vi "Any_Ref_enthalpy_funct_PS_REFPROP10.vi"(1 "Pressure Out (kPa)":dbl, 2 "S_in":dbl, 3 "error in (no error)":errorcluster, 4 "Fluidofinterest":string="R134a.FLD", 5 "?":path=path "C:/Users/ASITest/Desktop/REFPROP") -> (8 "h2_s":dbl, 10 "error out":errorcluster)   [LabVIEW 2016]
doc: "Return refrigerant enthalpy [kJ/kg] for specified refrigerant, input pressure [kPa] and temperature [C]"
panel:
  out "name out":string
  out "data":string[][](table)=[["0", "T", "40.917420"], ["1", "P", "632.917420"], ["2", "H", "466.332574"], ["3", "S", "2.054657"], ["4", "DV", "18.926081"], ["5", "DL", "18.926081"], ["6", "E", "432.891028"], ["7", "CV", "0.758226"], ["8", "CP", "0.924261"], ["9", "W", "194.299169"], ["10", "Q", "998.000000"]]
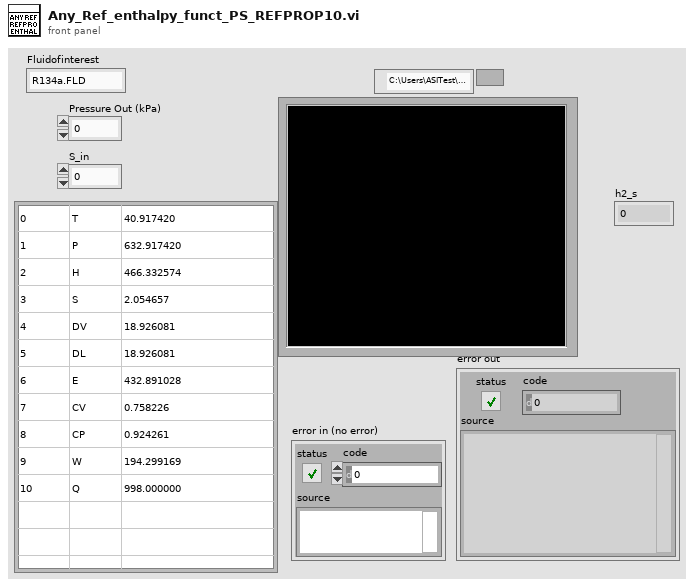
[diagram p1: front panel]
types:
  T1 = enum16{"0", "PS", "HS", "T", "P", "TP", "TH", "TS", "PH", "PQ", "TQ"}
  T2 = typedef "Mixture Composition cluster_d.ctl" = cluster{"Mixture Name":string, "Molecular weight (g/mol)":dbl, "Critical temperature (K)":dbl, "Critical Pressure (kPa)":dbl, "Critical Density (mol/L)":dbl, "# Components":i32, "Fluid File Paths":path[], "Component molar fractions":dbl[], "Refprop Main Directory":path, "DLL Version Number":dbl}
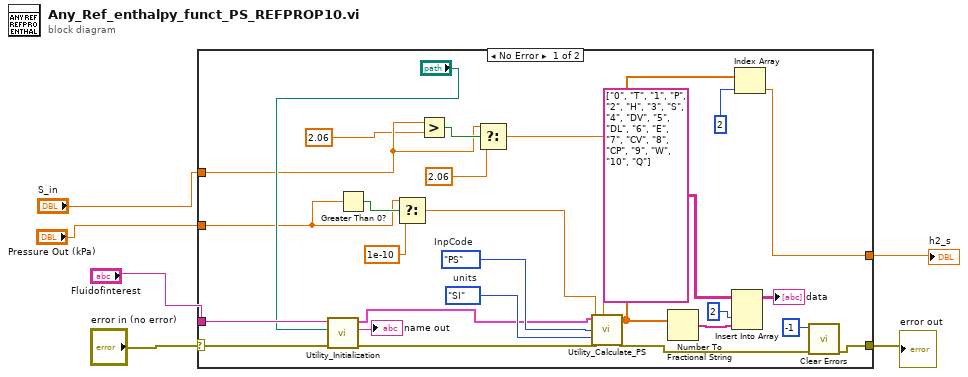
[diagram p0: block diagram]
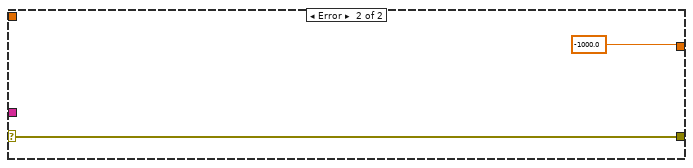
[diagram p2: hidden frame]
diagram:
  n1 = case shown="No Error" "error in (no error)" {
    selector: "error in (no error)" -> [w29 w35]
    tunnel: [w27 w35] -> w5
    tunnel: "S_in" -> [w8 _]
    tunnel: "Fluidofinterest" -> [w28 _]
    tunnel: "Pressure Out (kPa)" -> [w14 _]
    tunnel: [w24 -1000.0 ("Numeric")] -> w3
    frame No Error {
      w21 = T1."PS"  # InpCode
      w22 = enum16{"SI", "IP"}."SI"  # units
      n2 = call "Utility_Initialization.vi"("error in (no error)"=w29, "path"="?", "Fluidofinterest"=w28) -> ("error out"=w23:errorcluster, "name out"=→"name out":string, "Mixure Cluster out"=w20:T2)  [unwired: 6 in]
      n3 = Greater Than 0?(x=w14) -> (x > 0?=w15:bool)
      n4 = Select(t=w14, s=w15, f=1e-10) -> (s? t:f=w12:dbl)
      n5 = Greater?(x=w8, y=2.06) -> (0:w11:bool)
      n6 = Select(t=w8, s=w11, f=2.06) -> (s? t:f=w9:dbl)
      n7 = call "Utility_Calculate_PS.vi"("input_2"=w9, "input_1"=w12, "error in"=w23, "units"=w22, "InpCode"=w21, "Mixure Cluster"=w20) -> ("error out"=w19:errorcluster, "dataout"=w17:dbl[])  [unwired: 3 in, 1 out]
      n8 = Number To Fractional String(number=w17) -> (F-format string=w18:string[])  [unwired: 3 in]
      n9 = Insert Into Array(array=string[][] [["0", "T"], ["1", "P"], ["2", "H"], ["3", "S"], ["4", "DV"], ["5", "DL"], ["6", "E"], ["7", "CV"], ["8", "CP"], ["9", "W"], ["10", "Q"]] ("数组"), index (col)=2 ("禁用的索引 (列)"), new element=w18) -> (→"data":string[][])  [unwired: 1 in]
      n10 = Index Array(array=w17, index=2) -> (element=w24:dbl)
      n11 = call <vilib>:"Clear Errors.vi"("error in (no error)"=w19, "specific error code to clear (0: all)"=-1) -> ("error out"=w27:errorcluster)  [unwired: 4 in, 1 out]
    }
    frame Error {
    }
  }
  "error out" <- w5
  "h2_s" <- w3
